vi "Core.vi"() -> (19 "Error Out":errorcluster)   [LabVIEW 2017]
uses:
  <vilib>/Platform/TimedLoop/XDataNode/timing_clust.ctl
  <vilib>/Platform/TimedLoop/XDataNode/nitl_modes.ctl
  <vilib>/Platform/TimedLoop/XDataNode/wakeup.ctl
  <vilib>/Platform/TimedLoop/XDataNode/XDataNode.xnode
  <vilib>/Platform/TimedLoop/XDataNode/XDNodeRunTimeDep.lvlib
panel:
  in  "Shutdown":bool
  out "Output Resistance":dbl
  # "Core Module DIagnostics"
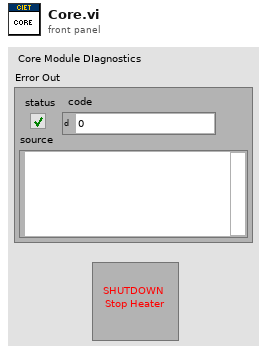
[diagram p1: front panel]
types:
  T1 = typedef "XDNodeRunTimeDep.lvlib/timing_clust.ctl" = cluster{"Expected End [f-1]":u64, "Actual End [f-1]":u64, "Finished Late? [f-1]":bool, "Expected End [i-1]":u64, "Actual End [i-1]":u64, "Finished Late? [i-1]":bool, "Expected Start [i]":u64, "Actual Start [i]":u64, "Expected Start [f]":u64, "Actual Start [f]":u64, "Source Name":string, "Structure Name":string, "Period":i64, "Deadline":i64, "Offset":i64, "Start":i64, "Priority":i32, "Timeout":i32, "Mode":T2, "Wakeup Reason":T3, "Error":errorcluster, "Source Type":string, "Secondary Source Type":string, "Global End Time":u64, "Global Start Time":u64, "Frame Duration":u64, "Iteration Duration":u64, "Assigned CPU":i32, "I/O Scan Engine Mode":u32}
  T2 = typedef "XDNodeRunTimeDep.lvlib/nitl_modes.ctl" = enum32{"No Change", "Process missed periods, maintain original phase", "Discard missed periods, maintain original phase", "Process missed periods, ignore original phase", "Discard missed periods, ignore original phase"}
  T3 = typedef "XDNodeRunTimeDep.lvlib/wakeup.ctl" = enum32{"Normal", "Aborted", "Asynchronous wakeup", "Timing source error", "Timed loop error", "Timeout"}
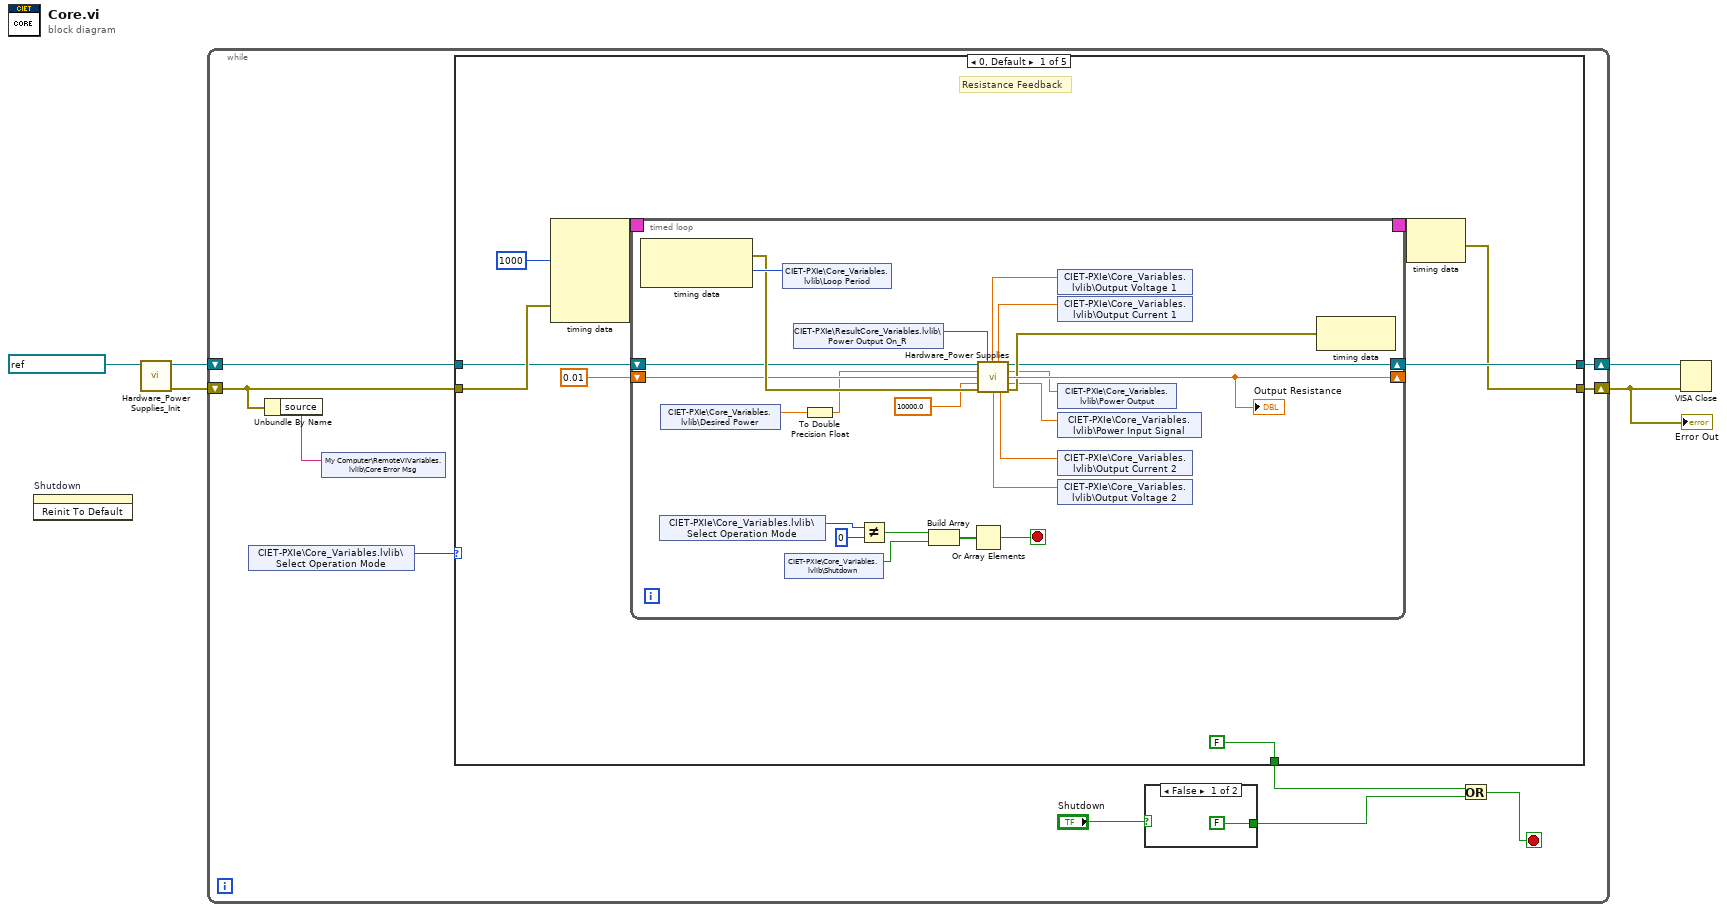
[diagram p0: block diagram]
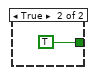
[diagram p2: hidden frame]
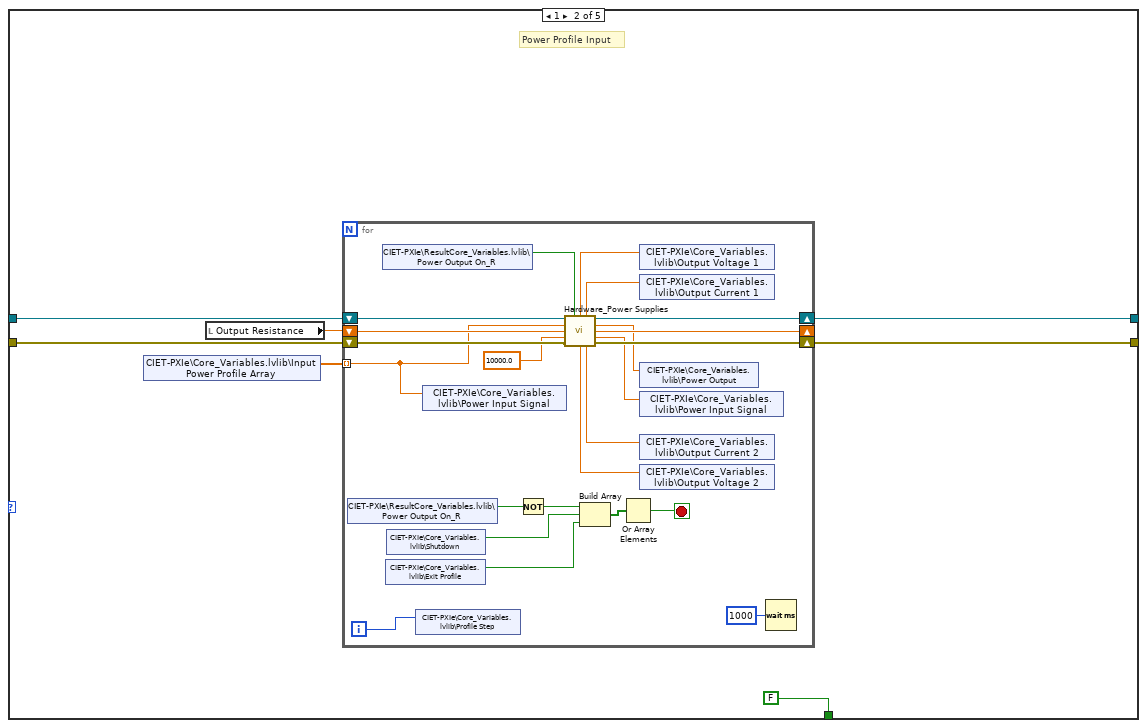
[diagram p3: hidden frame]
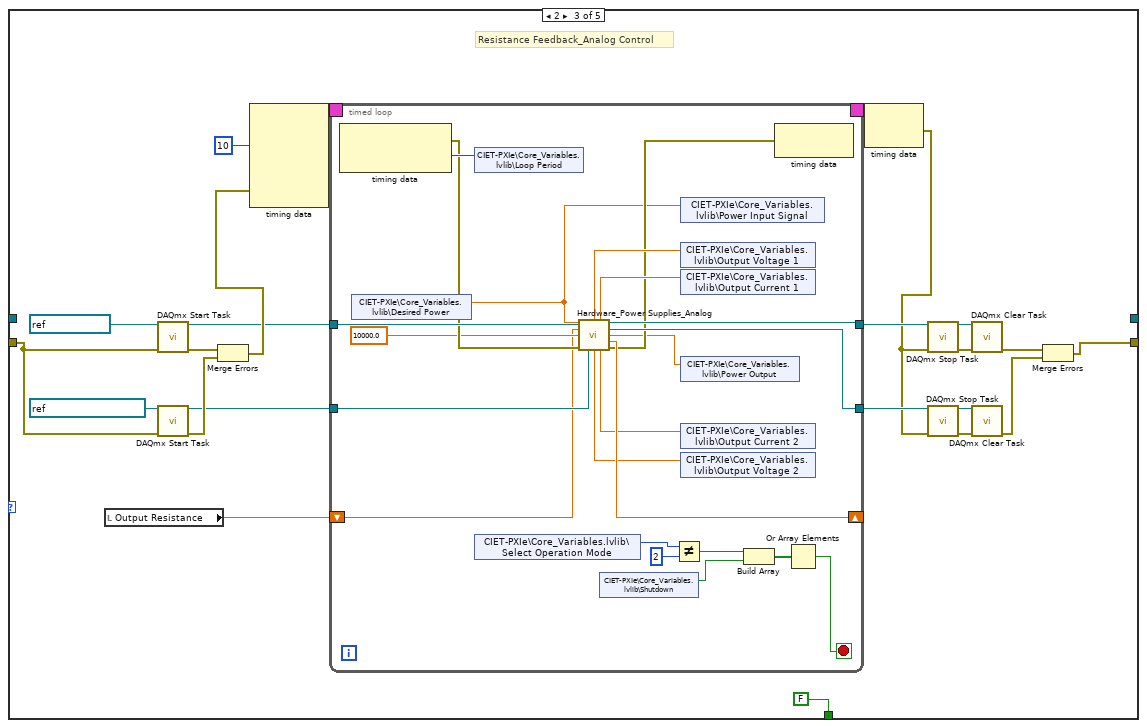
[diagram p4: hidden frame]
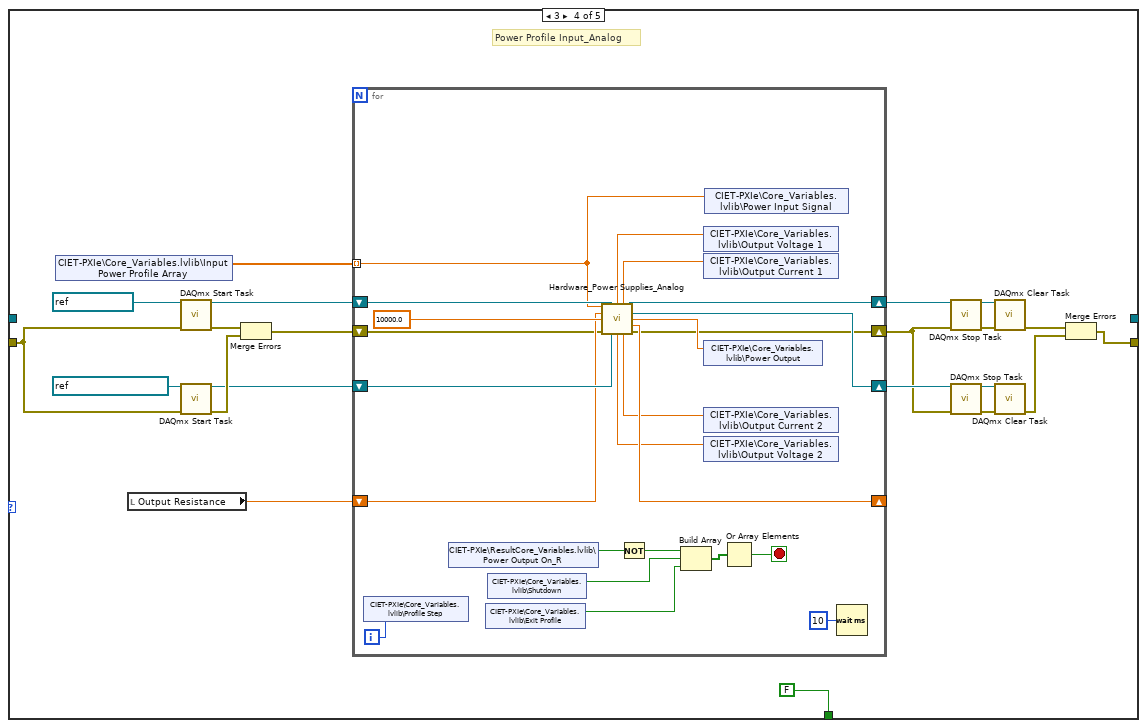
[diagram p5: hidden frame]
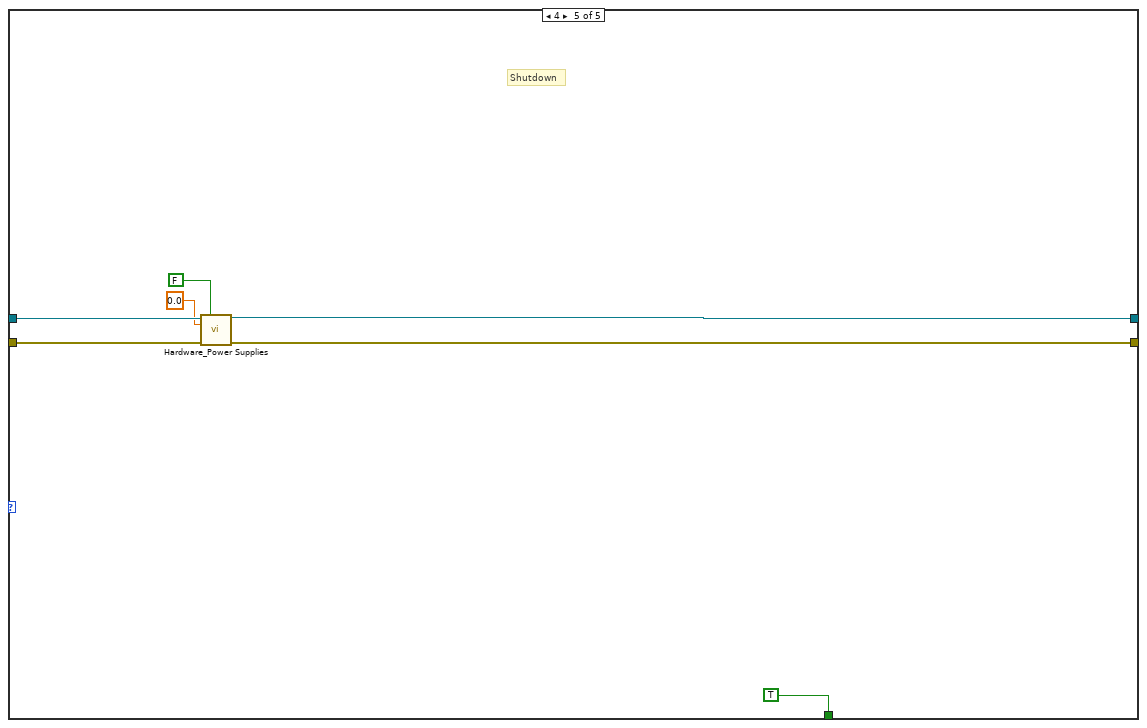
[diagram p6: hidden frame]
diagram:
  n1 = invoke on="Shutdown" class="Bool (strict)" method="Reinit To Default"() -> ()  [unwired: 3 in, 3 out]
  n2 = call "Hardware_Power Supplies_Init.vi"("VISA name"=refnum<visa-resource-name> "PowerSupply") -> ("Error out"=w1:errorcluster, "VISA out"=w2:refnum<visa-resource-name>)  [unwired: 9 in]
  n3 = while {
    shift-right: [w13] -> w4
    shift-left: w1 -> [w7]
    shift-right: [w14] -> w5
    shift-left: w2 -> [w15]
    stop <- w9 stop-if-true
    n4 = shared-variable "CIET-PXIe\\Core_Variables.lvlib\\Select Operation Mode"() -> (w12:u16)  [unwired: 1 in, 1 out]
    n5 = Unbundle By Name(w7) -> ("source"=w6:string)
    n6 = shared-variable "My Computer\\RemoteVIVariables.lvlib\\Core Error Msg"(w6) -> ()  [unwired: 1 in, 1 out]
    n7 = case shown="0, Default" w12 {
      tunnel: w7 -> [w24 w65 w99 w154 w198]
      tunnel: w15 -> [w23 w68 _ _ w197]
      tunnel: [w21 w67 _ _ w196] -> w14
      tunnel: [w20 w64 w104 w153 w195] -> w13
      tunnel: [FALSE ("Shutdown") FALSE ("Shutdown") FALSE ("Shutdown") FALSE ("Shutdown") TRUE ("Shutdown")] -> w11
      frame 0, Default {
        # "Resistance Feedback"
        n8 = node-c288(i64 1000 ("Period"), w24) -> (w26:T1)  [unwired: 3 in]
        n9 = timed-loop {
          timing: w26 -> [_]
          timing-out: [_] -> w25
          shift-right: [w34] -> w21
          shift-left: w23 -> [w41]
          shift-right: [w38] -> _
          shift-left: 0.01 -> [w40]
          stop <- w46 stop-if-true
          n10 = node-c288() -> (w42:errorcluster, w45:i64)  [unwired: 1 in]
          n11 = shared-variable "CIET-PXIe\\Core_Variables.lvlib\\Select Operation Mode"() -> (w44:u16)  [unwired: 1 in, 1 out]
          n12 = shared-variable "CIET-PXIe\\Core_Variables.lvlib\\Desired Power"() -> (w28:sgl)  [unwired: 1 in, 1 out]
          n13 = shared-variable "CIET-PXIe\\Core_Variables.lvlib\\Loop Period"(w45) -> ()  [unwired: 1 in, 1 out]
          n14 = shared-variable "CIET-PXIe\\Core_Variables.lvlib\\Shutdown"() -> (w43:bool)  [unwired: 1 in, 1 out]
          n15 = shared-variable "CIET-PXIe\\ResultCore_Variables.lvlib\\Power Output On_R"() -> (w33:bool)  [unwired: 1 in, 1 out]
          n16 = To Double Precision Float(number=w28) -> (double precision float=w27:dbl)
          n17 = Not Equal?(x=w44, y=u16 0) -> (x != y?=w48:bool)
          n18 = Build Array(w48, w43) -> (w47:bool[])
          n19 = Or Array Elements(Boolean array=w47) -> (logical OR=w46:bool)
          n20 = call "Hardware_Power Supplies.vi"("Input VISA"=w41, "Power Output ON"=w33, "Desired Power"=w27, "Input Resistance"=w40, "Maximum Power Limit"=10000.0, "Input Error"=w42) -> ("Output Voltage 1"=w32:dbl, "Output Current 1"=w31:dbl, "Output VISA"=w34:refnum<visa-resource-name>, "Output Power"=w35:dbl, "Output Resistance"=w38:dbl, "Input Power"=w36:dbl, "Output Voltage 2"=w29:dbl, "Output Current 2"=w30:dbl, "Output Error"=w37:errorcluster)  [unwired: 1 in]
          "Output Resistance" <- w38
          n21 = shared-variable "CIET-PXIe\\Core_Variables.lvlib\\Output Voltage 1"(w32) -> ()  [unwired: 1 in, 1 out]
          n22 = shared-variable "CIET-PXIe\\Core_Variables.lvlib\\Output Current 1"(w31) -> ()  [unwired: 1 in, 1 out]
          n23 = shared-variable "CIET-PXIe\\Core_Variables.lvlib\\Power Output"(w35) -> ()  [unwired: 1 in, 1 out]
          n24 = shared-variable "CIET-PXIe\\Core_Variables.lvlib\\Power Input Signal"(w36) -> ()  [unwired: 1 in, 1 out]
          n25 = shared-variable "CIET-PXIe\\Core_Variables.lvlib\\Output Current 2"(w30) -> ()  [unwired: 1 in, 1 out]
          n26 = shared-variable "CIET-PXIe\\Core_Variables.lvlib\\Output Voltage 2"(w29) -> ()  [unwired: 1 in, 1 out]
          n27 = node-c288(w37) -> ()  [unwired: 1 out]
        }
        n28 = node-c288(w25) -> (w20:errorcluster)
      }
      frame 1 {
        # "Power Profile Input"
        n29 = shared-variable "CIET-PXIe\\Core_Variables.lvlib\\Input Power Profile Array"() -> (w62:dbl[])  [unwired: 1 in, 1 out]
        n30 = local read "Output Resistance"() -> (w66:dbl)
        n31 = for {
          shift-right: [w83] -> w67
          shift-left: w68 -> [w84]
          shift-right: [w82] -> w64
          shift-left: w65 -> [w81]
          tunnel: w62 -> [w69] mode=indexing
          shift-right: [w75] -> _
          shift-left: w66 -> [w74]
          i -> [w85]
          stop <- w89 stop-if-true
          n32 = shared-variable "CIET-PXIe\\ResultCore_Variables.lvlib\\Power Output On_R"() -> (w87:bool)  [unwired: 1 in, 1 out]
          n33 = shared-variable "CIET-PXIe\\ResultCore_Variables.lvlib\\Power Output On_R"() -> (w80:bool)  [unwired: 1 in, 1 out]
          n34 = shared-variable "CIET-PXIe\\Core_Variables.lvlib\\Exit Profile"() -> (w70:bool)  [unwired: 1 in, 1 out]
          n35 = shared-variable "CIET-PXIe\\Core_Variables.lvlib\\Shutdown"() -> (w86:bool)  [unwired: 1 in, 1 out]
          n36 = shared-variable "CIET-PXIe\\Core_Variables.lvlib\\Profile Step"(w85) -> ()  [unwired: 1 in, 1 out]
          n37 = shared-variable "CIET-PXIe\\Core_Variables.lvlib\\Power Input Signal"(w69) -> ()  [unwired: 1 in, 1 out]
          n38 = Not(x=w87) -> (.not. x?=w88:bool)
          n39 = call "Hardware_Power Supplies.vi"("Input VISA"=w84, "Power Output ON"=w80, "Desired Power"=w69, "Input Resistance"=w74, "Maximum Power Limit"=10000.0, "Input Error"=w81) -> ("Output Voltage 1"=w79:dbl, "Output Current 1"=w78:dbl, "Output VISA"=w83:refnum<visa-resource-name>, "Output Power"=w72:dbl, "Output Resistance"=w75:dbl, "Input Power"=w71:dbl, "Output Voltage 2"=w77:dbl, "Output Current 2"=w76:dbl, "Output Error"=w82:errorcluster)  [unwired: 1 in]
          n40 = Build Array(w88, w86, w70) -> (w91:bool[])
          n41 = Or Array Elements(Boolean array=w91) -> (logical OR=w89:bool)
          n42 = shared-variable "CIET-PXIe\\Core_Variables.lvlib\\Output Voltage 1"(w79) -> ()  [unwired: 1 in, 1 out]
          n43 = shared-variable "CIET-PXIe\\Core_Variables.lvlib\\Output Current 1"(w78) -> ()  [unwired: 1 in, 1 out]
          n44 = shared-variable "CIET-PXIe\\Core_Variables.lvlib\\Power Output"(w72) -> ()  [unwired: 1 in, 1 out]
          n45 = shared-variable "CIET-PXIe\\Core_Variables.lvlib\\Power Input Signal"(w71) -> ()  [unwired: 1 in, 1 out]
          n46 = shared-variable "CIET-PXIe\\Core_Variables.lvlib\\Output Current 2"(w76) -> ()  [unwired: 1 in, 1 out]
          n47 = shared-variable "CIET-PXIe\\Core_Variables.lvlib\\Output Voltage 2"(w77) -> ()  [unwired: 1 in, 1 out]
          n48 = Wait (ms)(milliseconds to wait=u32 1000) -> ()  [unwired: 1 out]
        }
      }
      frame 2 {
        # "Resistance Feedback_Analog Control"
        n49 = local read "Output Resistance"() -> (w96:dbl)
        n50 = call <vilib>:"DAQmx Start Task.vi"("task/channels in"=refnum<k21> "PowerOut", "error in"=w99) -> ("task out"=w98:refnum<k21>, "error out"=w114:errorcluster)  [unwired: 12 in]
        n51 = call <vilib>:"DAQmx Start Task.vi"("task/channels in"=refnum<k21> "PowerMonitor_V", "error in"=w99) -> ("task out"=w97:refnum<k21>, "error out"=w113:errorcluster)  [unwired: 12 in]
        n52 = Merge Errors(w114, w113) -> (w100:errorcluster)
        n53 = node-c288(i64 10 ("Period"), w100) -> (w103:T1)  [unwired: 3 in]
        n54 = timed-loop {
          timing: w103 -> [_]
          timing-out: [_] -> w102
          shift-right: [w130] -> _
          shift-left: w96 -> [w131]
          tunnel: w98 -> [w135]
          tunnel: [w129] -> w95
          tunnel: w97 -> [w134]
          tunnel: [w128] -> w94
          stop <- w116 stop-if-true
          n55 = node-c288() -> (w133:errorcluster, w136:i64)  [unwired: 1 in]
          n56 = shared-variable "CIET-PXIe\\Core_Variables.lvlib\\Desired Power"() -> (w115:sgl)  [unwired: 1 in, 1 out]
          n57 = shared-variable "CIET-PXIe\\Core_Variables.lvlib\\Loop Period"(w136) -> ()  [unwired: 1 in, 1 out]
          n58 = shared-variable "CIET-PXIe\\Core_Variables.lvlib\\Select Operation Mode"() -> (w118:u16)  [unwired: 1 in, 1 out]
          n59 = call "Hardware_Power Supplies_Analog.vi"("Desired Power"=w115, "Task In_1"=w135, "Input Resistance"=w131, "Maximum Power Limit"=10000.0, "Error In"=w133, "Task In_2"=w134) -> ("Output Voltage 1"=w127:dbl, "Output Current 1"=w126:dbl, "Task Out_1"=w129:refnum<k21>, "Task Out_2"=w128:refnum<k21>, "Output Power"=w122:dbl, "Output Resistance"=w130:dbl, "Output Voltage 2"=w125:dbl, "Output Current 2"=w124:dbl, "Error Out"=w123:errorcluster)  [unwired: 1 in]
          n60 = shared-variable "CIET-PXIe\\Core_Variables.lvlib\\Shutdown"() -> (w117:bool)  [unwired: 1 in, 1 out]
          n61 = Not Equal?(x=w118, y=u16 2) -> (x != y?=w120:bool)
          n62 = shared-variable "CIET-PXIe\\Core_Variables.lvlib\\Power Input Signal"(w115) -> ()  [unwired: 1 in, 1 out]
          n63 = shared-variable "CIET-PXIe\\Core_Variables.lvlib\\Output Voltage 1"(w127) -> ()  [unwired: 1 in, 1 out]
          n64 = shared-variable "CIET-PXIe\\Core_Variables.lvlib\\Output Current 1"(w126) -> ()  [unwired: 1 in, 1 out]
          n65 = shared-variable "CIET-PXIe\\Core_Variables.lvlib\\Power Output"(w122) -> ()  [unwired: 1 in, 1 out]
          n66 = shared-variable "CIET-PXIe\\Core_Variables.lvlib\\Output Current 2"(w124) -> ()  [unwired: 1 in, 1 out]
          n67 = shared-variable "CIET-PXIe\\Core_Variables.lvlib\\Output Voltage 2"(w125) -> ()  [unwired: 1 in, 1 out]
          n68 = Build Array(w120, w117) -> (w119:bool[])
          n69 = node-c288(w123) -> ()  [unwired: 1 out]
          n70 = Or Array Elements(Boolean array=w119) -> (logical OR=w116:bool)
        }
        n71 = node-c288(w102) -> (w92:errorcluster)
        n72 = call <vilib>:"DAQmx Stop Task.vi"("task/channels in"=w95, "error in"=w92) -> ("task out"=w110:refnum<k21>, "error out"=w109:errorcluster)  [unwired: 12 in]
        n73 = call <vilib>:"DAQmx Stop Task.vi"("task/channels in"=w94, "error in"=w92) -> ("task out"=w108:refnum<k21>, "error out"=w107:errorcluster)  [unwired: 12 in]
        n74 = call <vilib>:"DAQmx Clear Task.vi"("task in"=w110, "error in"=w109) -> ("error out"=w106:errorcluster)  [unwired: 13 in]
        n75 = call <vilib>:"DAQmx Clear Task.vi"("task in"=w108, "error in"=w107) -> ("error out"=w105:errorcluster)  [unwired: 13 in]
        n76 = Merge Errors(w106, w105) -> (w104:errorcluster)
      }
      frame 3 {
        # "Power Profile Input_Analog"
        n77 = shared-variable "CIET-PXIe\\Core_Variables.lvlib\\Input Power Profile Array"() -> (w150:dbl[])  [unwired: 1 in, 1 out]
        n78 = local read "Output Resistance"() -> (w157:dbl)
        n79 = call <vilib>:"DAQmx Start Task.vi"("task/channels in"=refnum<k21> "PowerOut", "error in"=w154) -> ("task out"=w159:refnum<k21>, "error out"=w169:errorcluster)  [unwired: 12 in]
        n80 = call <vilib>:"DAQmx Start Task.vi"("task/channels in"=refnum<k21> "PowerMonitor_V", "error in"=w154) -> ("task out"=w158:refnum<k21>, "error out"=w168:errorcluster)  [unwired: 12 in]
        n81 = Merge Errors(w169, w168) -> (w152:errorcluster)
        n82 = for {
          shift-right: [w188] -> _
          shift-left: w157 -> [w189]
          shift-right: [w187] -> w156
          shift-left: w159 -> [w192]
          shift-right: [w186] -> w155
          shift-left: w158 -> [w191]
          shift-right: [w179] -> w151
          shift-left: w152 -> [w180]
          tunnel: w150 -> [w170] mode=indexing
          i -> [w174]
          stop <- w173 stop-if-true
          n83 = shared-variable "CIET-PXIe\\Core_Variables.lvlib\\Profile Step"(w174) -> ()  [unwired: 1 in, 1 out]
          n84 = shared-variable "CIET-PXIe\\ResultCore_Variables.lvlib\\Power Output On_R"() -> (w176:bool)  [unwired: 1 in, 1 out]
          n85 = shared-variable "CIET-PXIe\\Core_Variables.lvlib\\Exit Profile"() -> (w171:bool)  [unwired: 1 in, 1 out]
          n86 = shared-variable "CIET-PXIe\\Core_Variables.lvlib\\Shutdown"() -> (w175:bool)  [unwired: 1 in, 1 out]
          n87 = call "Hardware_Power Supplies_Analog.vi"("Desired Power"=w170, "Task In_1"=w192, "Input Resistance"=w189, "Maximum Power Limit"=10000.0, "Error In"=w180, "Task In_2"=w191) -> ("Output Voltage 1"=w185:dbl, "Output Current 1"=w184:dbl, "Task Out_1"=w187:refnum<k21>, "Task Out_2"=w186:refnum<k21>, "Output Power"=w181:dbl, "Output Resistance"=w188:dbl, "Output Voltage 2"=w183:dbl, "Output Current 2"=w182:dbl, "Error Out"=w179:errorcluster)  [unwired: 1 in]
          n88 = Not(x=w176) -> (.not. x?=w177:bool)
          n89 = Build Array(w177, w175, w171) -> (w178:bool[])
          n90 = shared-variable "CIET-PXIe\\Core_Variables.lvlib\\Output Voltage 1"(w185) -> ()  [unwired: 1 in, 1 out]
          n91 = shared-variable "CIET-PXIe\\Core_Variables.lvlib\\Output Current 1"(w184) -> ()  [unwired: 1 in, 1 out]
          n92 = shared-variable "CIET-PXIe\\Core_Variables.lvlib\\Power Output"(w181) -> ()  [unwired: 1 in, 1 out]
          n93 = shared-variable "CIET-PXIe\\Core_Variables.lvlib\\Output Current 2"(w182) -> ()  [unwired: 1 in, 1 out]
          n94 = shared-variable "CIET-PXIe\\Core_Variables.lvlib\\Output Voltage 2"(w183) -> ()  [unwired: 1 in, 1 out]
          n95 = shared-variable "CIET-PXIe\\Core_Variables.lvlib\\Power Input Signal"(w170) -> ()  [unwired: 1 in, 1 out]
          n96 = Or Array Elements(Boolean array=w178) -> (logical OR=w173:bool)
          n97 = Wait (ms)(milliseconds to wait=u32 10) -> ()  [unwired: 1 out]
        }
        n98 = call <vilib>:"DAQmx Stop Task.vi"("task/channels in"=w156, "error in"=w151) -> ("task out"=w165:refnum<k21>, "error out"=w164:errorcluster)  [unwired: 12 in]
        n99 = call <vilib>:"DAQmx Stop Task.vi"("task/channels in"=w155, "error in"=w151) -> ("task out"=w163:refnum<k21>, "error out"=w162:errorcluster)  [unwired: 12 in]
        n100 = call <vilib>:"DAQmx Clear Task.vi"("task in"=w165, "error in"=w164) -> ("error out"=w161:errorcluster)  [unwired: 13 in]
        n101 = call <vilib>:"DAQmx Clear Task.vi"("task in"=w163, "error in"=w162) -> ("error out"=w160:errorcluster)  [unwired: 13 in]
        n102 = Merge Errors(w161, w160) -> (w153:errorcluster)
      }
      frame 4 {
        # "Shutdown"
        n103 = call "Hardware_Power Supplies.vi"("Input VISA"=w197, "Power Output ON"=FALSE, "Desired Power"=0.0, "Input Error"=w198) -> ("Output VISA"=w196:refnum<visa-resource-name>, "Output Error"=w195:errorcluster)  [unwired: 3 in, 7 out]
      }
    }
    n104 = case shown="False" "Shutdown" {
      tunnel: [FALSE ("Shutdown") TRUE ("Shutdown")] -> w10
      frame False {
      }
      frame True {
      }
    }
    n105 = Or(x=w11, y=w10) -> (x .or. y?=w9:bool)
  }
  "Error Out" <- w4
  n106 = VISA Close(VISA resource name=w5, error in (no error)=w4) -> ()  [unwired: 1 out]
